vi "2013_02_18 Pre-Clinical Main jace laptop.vi"() -> ()   [LabVIEW 2012]
uses:
  Pre-Clinical Type Def.ctl
  <vilib>/DAQmx/write.llb/DAQmx Write (Analog 1D DBL NChan 1Samp).vi
  <vilib>/DAQmx/write.llb/DAQmx Write (Counter Time 1Chan 1Samp).vi
  <vilib>/DAQmx/read.llb/DAQmx Read (Analog 1D Wfm NChan NSamp).vi
  <vilib>/DAQmx/miscellaneous.llb/DAQmx Fill In Error Info.vi
  <resource>/objmgr/daqmx.rc
panel:
  out "Error":bool
  out "XY Graph 3":cluster{"Array":dbl[], "Array":dbl[]}[](graph)
  in  "X axis":u16(ring)=5 items=["Elapsed Time (s)"=0, "Source Current (A)"=10, "Supply (V)"=4, "Supply Power (W)"=11, "RMS Current (A) 1"=1, "RMS Voltage (V) 1"=2, "Electrical Power (W)"=6, "ESC Efficiency (%)"=12, "Torque (mNm)"=5, "RPM"=3, "Mechanical Power(W)"=7, "Motor Efficiency (%)"=8]
  in  "Capture":bool=TRUE
  in  "Y axis":u16(ring)=3 items=["Elapsed Time (s)"=0, "Source Current (A)"=10, "Supply (V)"=4, "Supply Power (W)"=11, "RMS Current (A) 1"=1, "RMS Voltage (V) 1"=2, "Electrical Power (W)"=6, "ESC Efficiency (%)"=12, "Torque (mNm)"=5, "RPM"=3, "Mechanical Power(W)"=7, "Motor Efficiency (%)"=8]
  out "TotalSampPerChanAcquired":dbl
  out "AvailSampPerChan":u32
  out "XY Graph 2":cluster{"Array":dbl[], "Array":dbl[]}[](graph)
  out "Single Motor 2":waveform(dbl)[](graph)
  in  "Waveform":bool
  out "XY Graph":cluster{"Array":dbl[], "Array":dbl[]}(graph)
  out "error out":errorcluster
  in  "File Path":path=path "C:/Users/Bullpen/Dropbox/Procyrion/Quality System/Hardware/Motors/Quality Results/.lvm"
  in  "Motor 1":T1 {"ESC Efficiency" format="%#_3g%%"; "Supply Power (W)" format="%.3f"; "Mechanical Power (W)" format="%.3f"; "Motor Efficiency" format="%#_3g%%"; "Electrical Power (W)" format="%.3f"; "Torque (mNm)" format="%.3f"; "Elapsed Time" format="%<%H:%M:%S>t"; "Supply (V)" format="%.2f"; "RPM" scale=0.0..60000.0}
  out "loop time (ms)":u32
  in  "stop":bool
  in  "PWM 1":dbl(slide) min=0.0 max=100.0 step=5.0 scale=0.0..100.0
  # "Fail"
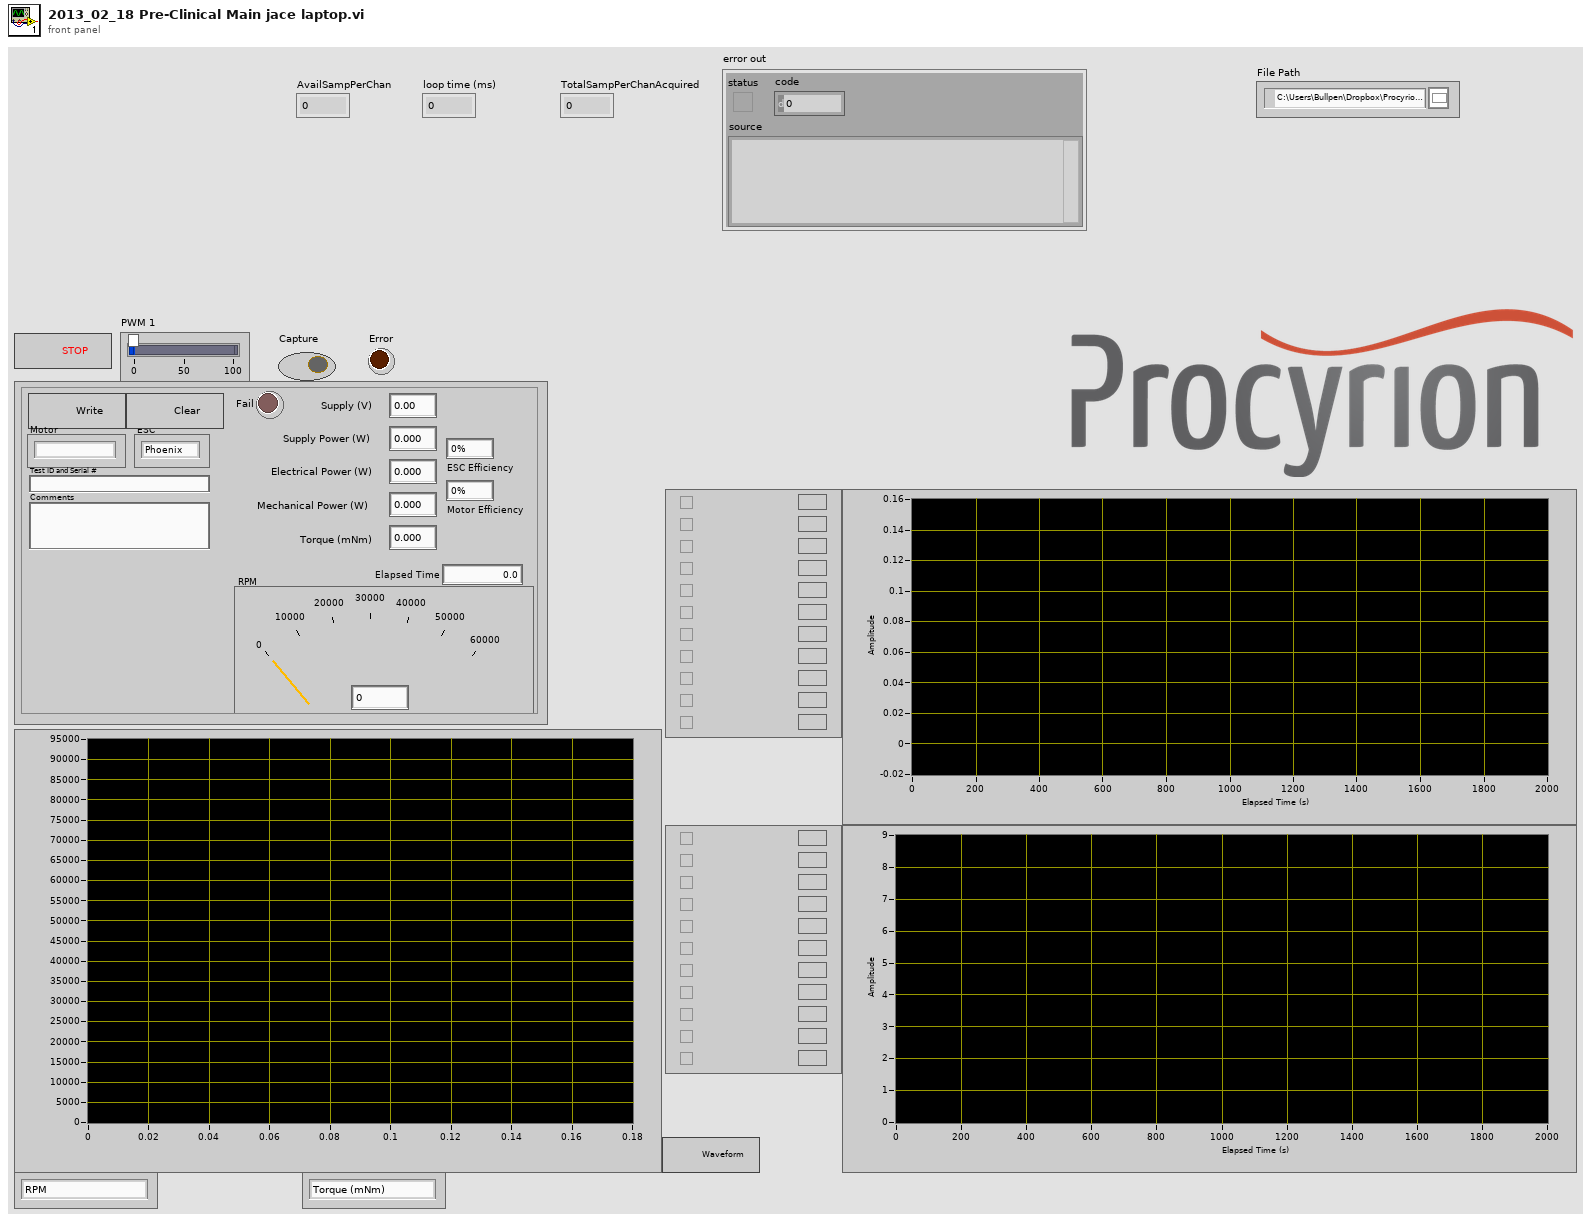
[diagram p1: front panel]
types:
  T1 = typedef "Pre-Clinical Type Def.ctl" = cluster{"Write":bool, "Fail":bool, "RPM":u64, "Motor":enum16{"", "Maxon EC6 6V", "Maxon EC4 6V", "FH 0620 6V", "FH 0620 12V", "FH 0427 6V K2540"}, "ESC":enum16{"Phoenix", "Maxon", "FH 1801"}, "Supply (V)":dbl, "Test ID and Serial #":string, "Comments":string, "Elapsed Time":dbl, "Counter":dbl, "Torque (mNm)":dbl, "Electrical Power (W)":dbl, "Motor Efficiency":dbl, "Mechanical Power (W)":dbl, "Supply Power (W)":dbl, "ESC Efficiency":dbl, "Clear":bool}
  T2 = enum16{"", "Maxon EC6 6V", "Maxon EC4 6V", "FH 0620 6V", "FH 0620 12V", "FH 0427 6V K2540"}
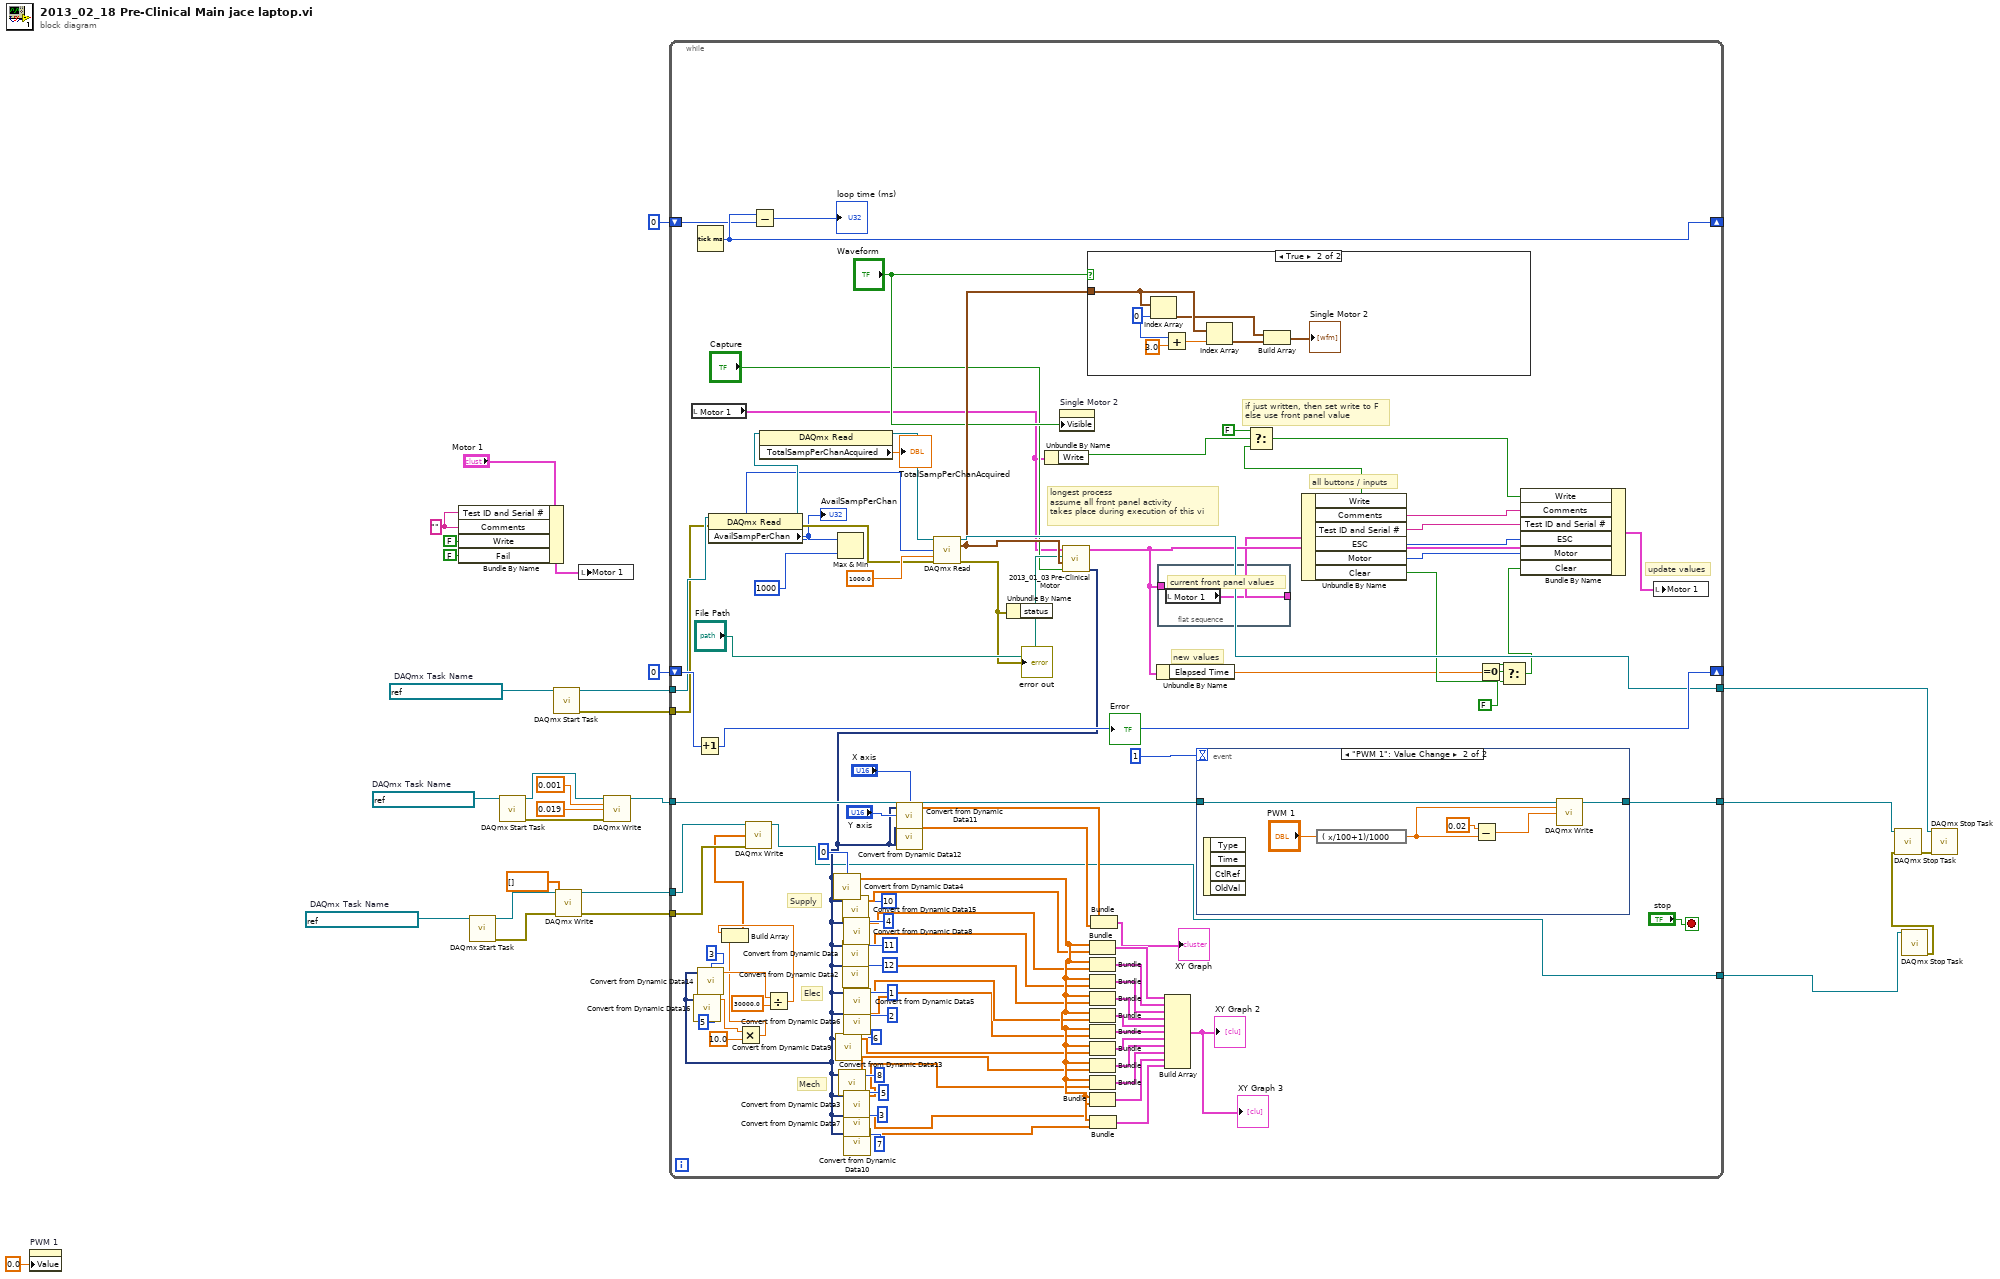
[diagram p0: block diagram]
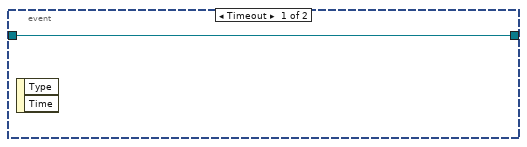
[diagram p3: hidden frame]
diagram:
  w8 = refnum<k21> "Pre-Clinical ADI Out"  # DAQmx Task Name
  w10 = "" ("Comments")
  w26 = refnum<k21> "Pre-Clinical PWM"  # DAQmx Task Name
  w9 = refnum<k21> "Pre-Clinical Acquire"  # DAQmx Task Name
  n1 = property on="PWM 1" class="Slide (strict)"("Value"=0.0 ("PWM 1")) -> ()  [unwired: 2 in, 2 out]
  n2 = Bundle By Name(cluster="Motor 1", "Test ID and Serial #"=w10, "Comments"=w10, "Write"=FALSE ("Enabled"), "Fail"=FALSE) -> (w11:T1)
  n3 = call <vilib>:"DAQmx Start Task.vi"("task/channels in"=w8) -> ("task out"=w7:refnum<k21>, "error out"=w6:errorcluster)  [unwired: 13 in]
  n4 = call <vilib>:"DAQmx Start Task.vi"("task/channels in"=w26) -> ("task out"=w24:refnum<k21>, "error out"=w23:errorcluster)  [unwired: 13 in]
  n5 = call <vilib>:"DAQmx Start Task.vi"("task/channels in"=w9) -> ("task out"=w28:refnum<k21>, "error out"=w15:errorcluster)  [unwired: 13 in]
  n6 = call-poly <vilib>:"DAQmx Write.vi"("task/channels in"=w7, "data"=dbl[] [], "error in"=w6) -> ("task out"=w5:refnum<k21>, "error out"=w3:errorcluster)  [unwired: 10 in, 1 out]
  n7 = local write "Motor 1"(w11) -> ()
  n8 = call-poly <vilib>:"DAQmx Write.vi"("task/channels in"=w24, "high time"=0.001 ("data"), "low time"=0.019 ("data"), "error in"=w23) -> ("task out"=w25:refnum<k21>)  [unwired: 9 in, 2 out]
  n9 = while {
    tunnel: w28 -> [w98]
    tunnel: [w115] -> w27
    tunnel: w15 -> [w96]
    shift-right: [w123] -> _
    shift-left: u32 0 ("millisecond timer value") -> [w122]
    tunnel: w25 -> [w120]
    tunnel: [w119] -> w22
    shift-right: [w116] -> _
    shift-left: 0 ("for") -> [w117]
    tunnel: w5 -> [w45]
    tunnel: w3 -> [w37]
    tunnel: [w36] -> w2
    stop <- "stop" stop-if-true
    # "Mech"
    # "Elec"
    # "Supply"
    # "if just written, then set write to F\nelse use front panel value"
    # "all buttons / inputs"
    # "update values"
    # "new values"
    # "longest process\nassume all front panel activity\ntakes place during execution of this vi"
    n10 = local read "Motor 1"() -> (w44:T1)
    n11 = Increment(x=w117) -> (x+1=w116:i32)
    n12 = Tick Count (ms)() -> (millisecond timer value=w123:u32)
    n13 = property class="DAQmx Read"(reference=w98, error in=w96) -> (reference out=w94:refnum<k21>, error out=w95:errorcluster, "AvailSampPerChan"=w90:u32)
    "AvailSampPerChan" <- w90
    n14 = Subtract(x=w123, y=w122) -> (x-y=→"loop time (ms)":u32)
    n15 = property class="DAQmx Read"(reference=w94) -> (reference out=w93:refnum<k21>, "TotalSampPerChanAcquired"=→"TotalSampPerChanAcquired":dbl)  [unwired: 1 in, 1 out]
    n16 = Max & Min(x=w90, y=1000 ("number of samples per channel")) -> (max(x,y)=w89:u32)  [unwired: 1 out]
    n17 = call-poly <vilib>:"DAQmx Read.vi"("task/channels in"=w93, "number of samples per channel"=w89, "timeout"=1000.0, "error in"=w95) -> ("task out"=w115:refnum<k21>, "data"=w113:waveform(dbl)[], "error out"=w46:errorcluster)  [unwired: 9 in]
    "error out" <- w46
    n18 = Unbundle By Name(w46) -> ()  [unwired: 1 out]
    n19 = Unbundle By Name(w44) -> ("Write"=w74:bool)
    n20 = property on="Single Motor 2" class="WFGraph (strict)"("Visible"="Waveform") -> ()  [unwired: 2 in, 2 out]
    n21 = call "2013_01_03 Pre-Clinical Motor.vi"("Capture"="Capture", "data"=w113, "File Path"="File Path", "Motor Typedef"=w44) -> ("Final Out"=w40:dynamicdata, "Motor Typedef Out"=w80:T1)  [unwired: 6 in]
    n22 = call "Convert from Dynamic Data16"("Dynamic Data Type"=w40, "Channel"=5) -> ("Scalar"=w29:dbl)  [unwired: 2 in]
    n23 = call "Convert from Dynamic Data14"("Dynamic Data Type"=w40, "Channel"=3) -> ("Scalar"=w34:dbl)  [unwired: 2 in]
    n24 = Multiply(x=w29, y=10.0) -> (x*y=w30:dbl)
    n25 = Divide(x=w34, y=30000.0) -> (x/y=w33:dbl)
    n26 = Build Array(w33, w30) -> (w32:dbl[])
    n27 = call-poly <vilib>:"DAQmx Write.vi"("task/channels in"=w45, "data"=w32, "error in"=w37) -> ("task out"=w36:refnum<k21>)  [unwired: 10 in, 2 out]
    n28 = call "Convert from Dynamic Data4"("Dynamic Data Type"=w40, "Channel"=0) -> ("Array"=w70:dbl[])  [unwired: 2 in]
    n29 = call "Convert from Dynamic Data9"("Dynamic Data Type"=w40, "Channel"=6) -> ("Array"=w68:dbl[])  [unwired: 2 in]
    n30 = call "Convert from Dynamic Data13"("Dynamic Data Type"=w40, "Channel"=8) -> ("Array"=w48:dbl[])  [unwired: 2 in]
    n31 = call "Convert from Dynamic Data15"("Dynamic Data Type"=w40, "Channel"=10) -> ("Array"=w69:dbl[])  [unwired: 2 in]
    n32 = call "Convert from Dynamic Data"("Dynamic Data Type"=w40, "Channel"=11) -> ("Array"=w53:dbl[])  [unwired: 2 in]
    n33 = call "Convert from Dynamic Data2"("Dynamic Data Type"=w40, "Channel"=12) -> ("Array"=w52:dbl[])  [unwired: 2 in]
    n34 = call "Convert from Dynamic Data8"("Dynamic Data Type"=w40, "Channel"=4) -> ("Array"=w54:dbl[])  [unwired: 2 in]
    n35 = call "Convert from Dynamic Data3"("Dynamic Data Type"=w40, "Channel"=5) -> ("Array"=w42:dbl[])  [unwired: 2 in]
    n36 = call "Convert from Dynamic Data7"("Dynamic Data Type"=w40, "Channel"=3) -> ("Array"=w41:dbl[])  [unwired: 2 in]
    n37 = call "Convert from Dynamic Data5"("Dynamic Data Type"=w40, "Channel"=1) -> ("Array"=w51:dbl[])  [unwired: 2 in]
    n38 = call "Convert from Dynamic Data6"("Dynamic Data Type"=w40, "Channel"=2) -> ("Array"=w50:dbl[])  [unwired: 2 in]
    n39 = call "Convert from Dynamic Data10"("Dynamic Data Type"=w40, "Channel"=7) -> ("Array"=w49:dbl[])  [unwired: 2 in]
    n40 = call "Convert from Dynamic Data11"("Dynamic Data Type"=w40, "Channel"="X axis") -> ("Array"=w86:dbl[])  [unwired: 2 in]
    n41 = call "Convert from Dynamic Data12"("Dynamic Data Type"=w40, "Channel"="Y axis") -> ("Array"=w87:dbl[])  [unwired: 2 in]
    n42 = case shown="True" "Waveform" {
      tunnel: w113 -> [_ w130]
      frame False {
      }
      frame True {
        w131 = 0 ("index")
        n43 = Index Array(array=w130, index=w131) -> (element=w128:waveform(dbl))
        n44 = Add(x=w131, y=3.0) -> (x+y=w129:dbl)
        n45 = Index Array(array=w130, index=w129) -> (element=w127:waveform(dbl))
        n46 = Build Array(w128, w127) -> (→"Single Motor 2":waveform(dbl)[])
      }
    }
    n47 = Bundle("Array"=w70, "Array"=w69) -> (w102:cluster{"Array":dbl[], "Array":dbl[]})  [unwired: 1 in]
    n48 = Bundle("Array"=w70, "Array"=w54) -> (w103:cluster{"Array":dbl[], "Array":dbl[]})  [unwired: 1 in]
    n49 = Bundle("Array"=w70, "Array"=w53) -> (w104:cluster{"Array":dbl[], "Array":dbl[]})  [unwired: 1 in]
    n50 = Bundle("Array"=w70, "Array"=w52) -> (w105:cluster{"Array":dbl[], "Array":dbl[]})  [unwired: 1 in]
    n51 = Bundle("Array"=w70, "Array"=w51) -> (w106:cluster{"Array":dbl[], "Array":dbl[]})  [unwired: 1 in]
    n52 = Bundle("Array"=w70, "Array"=w50) -> (w107:cluster{"Array":dbl[], "Array":dbl[]})  [unwired: 1 in]
    n53 = Bundle("Array"=w70, "Array"=w68) -> (w108:cluster{"Array":dbl[], "Array":dbl[]})  [unwired: 1 in]
    n54 = Bundle("Array"=w70, "Array"=w48) -> (w109:cluster{"Array":dbl[], "Array":dbl[]})  [unwired: 1 in]
    n55 = Bundle("Array"=w70, "Array"=w42) -> (w111:cluster{"Array":dbl[], "Array":dbl[]})  [unwired: 1 in]
    n56 = Bundle("Array"=w70, "Array"=w41) -> (w110:cluster{"Array":dbl[], "Array":dbl[]})  [unwired: 1 in]
    n57 = Bundle("Array"=w70, "Array"=w49) -> (w100:cluster{"Array":dbl[], "Array":dbl[]})  [unwired: 1 in]
    n58 = Bundle("Array"=w86, "Array"=w87) -> (→"XY Graph":cluster{"Array":dbl[], "Array":dbl[]})  [unwired: 1 in]
    n59 = Unbundle By Name(w80) -> ("Elapsed Time"=w81:dbl)
    n60 = flat-sequence {
      tunnel: w80 -> [_]
      tunnel: [w125] -> w79
      frame #0 {
        # "current front panel values"
        n61 = local read "Motor 1"() -> (w125:T1)
      }
    }
    n62 = Build Array(w102, w103, w104, w105, w106, w107, w108, w109, w111, w110, w100) -> (→"XY Graph 2" →"XY Graph 3":cluster{"Array":dbl[], "Array":dbl[]}[])
    n63 = event shown="[1] \"PWM 1\": Value Change" {
      selector: _ -> [_ _]
      dyn-events: _ -> [_ _]
      timeout: 1 -> [_ _]
      tunnel: w120 -> [w133 w135]
      tunnel: [w133 w134] -> w119
      event Timeout {
        n64 = event-data() -> ()  [unwired: 1 in, 2 out]
      }
      event "PWM 1": Value Change {
        n65 = event-data() -> ()  [unwired: 1 in, 4 out]
        n66 = expression code="( x/100+1)/1000"("PWM 1") -> (w136:dbl)
        n67 = Subtract(x=0.02 ("y"), y=w136) -> (x-y=w137:dbl)
        n68 = call-poly <vilib>:"DAQmx Write.vi"("task/channels in"=w135, "high time"=w136, "low time"=w137) -> ("task out"=w134:refnum<k21>)  [unwired: 10 in, 2 out]
      }
    }
    n69 = Unbundle By Name(w79) -> ("Write"=w72:bool, "Comments"=w78:string, "Test ID and Serial #"=w77:string, "ESC"=w76:enum16{"Phoenix", "Maxon", "FH 1801"}, "Motor"=w75:T2, "Clear"=w83:bool)
    n70 = Select(t=FALSE, s=w74, f=w72) -> (s? t:f=w71:bool)
    n71 = Equal To 0?(x=w81) -> (x = 0?=w85:bool)
    n72 = Select(t=FALSE ("Calcul"), s=w85, f=w83) -> (s? t:f=w82:bool)
    n73 = Bundle By Name(cluster=w80, "Write"=w71, "Comments"=w78, "Test ID and Serial #"=w77, "ESC"=w76, "Motor"=w75, "Clear"=w82) -> (w114:T1)
    n74 = local write "Motor 1"(w114) -> ()
  }
  n75 = call <vilib>:"DAQmx Stop Task.vi"("task/channels in"=w2) -> ("error out"=w1:errorcluster)  [unwired: 13 in, 1 out]
  n76 = call <vilib>:"DAQmx Stop Task.vi"("task/channels in"=w22, "error in"=w1) -> ("error out"=w21:errorcluster)  [unwired: 12 in, 1 out]
  n77 = call <vilib>:"DAQmx Stop Task.vi"("task/channels in"=w27, "error in"=w21) -> ()  [unwired: 12 in, 2 out]
